vi "UpdateArray (SubVI).vi"(8 "log":bool, 9 "Temp1":dbl, 10 "Resolution":dbl, 11 "Array":dbl[](array[numeric])) -> (3 "x > y?":bool)   [LabVIEW 2014]
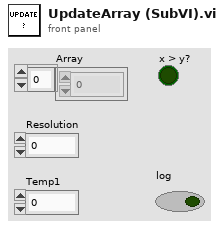
[diagram p1: front panel]
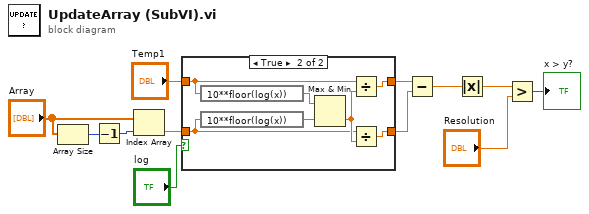
[diagram p0: block diagram]
diagram:
  n1 = Array Size(array="Array") -> (size(s)=w9:i32)
  n2 = Decrement(x=w9) -> (x-1=w10:i32)
  n3 = Index Array(array="Array", index=w10) -> (element=w4:dbl)
  n4 = case shown="True" "log" {
    tunnel: "Temp1" -> [w14 w18]
    tunnel: w4 -> [w13 w16]
    tunnel: [w14 w21] -> w3
    tunnel: [w13 w20] -> w2
    frame False {
    }
    frame True {
      n5 = expression code="10**floor(log(x))"(w18) -> (w17:dbl)
      n6 = expression code="10**floor(log(x))"(w16) -> (w15:dbl)
      n7 = Max & Min(x=w17, y=w15) -> (min(x,y)=w19:dbl)  [unwired: 1 out]
      n8 = Divide(x=w18, y=w19) -> (x/y=w21:dbl)
      n9 = Divide(x=w16, y=w19) -> (x/y=w20:dbl)
    }
  }
  n10 = Subtract(x=w3, y=w2) -> (x-y=w11:dbl)
  n11 = Absolute Value(x=w11) -> (abs(x)=w6:dbl)
  n12 = Greater?(x=w6, y="Resolution") -> (0:→"x > y?":bool)
